vi "this application info.vi"(8 "error in":errorcluster, 11 "Build Type":enum16{"Release", "Patch", "Beta"}(ring)=enum."Patch") -> (0 "error out":errorcluster, 1 "App Info":T1, 2 "FileVersion":string, 3 "Title":string)   [LabVIEW 2020, in "Reusable Library.lvlib"]
doc: "This VI will return the Version info of the exe during runtime environment."
uses:
  Reusable Library.lvlib
panel:
  # "VI Template By\n        Samuel James\n        Measurement Engineer\n        Certified LabVIEW Architect\n        Vestas Technology R&D Chennai"
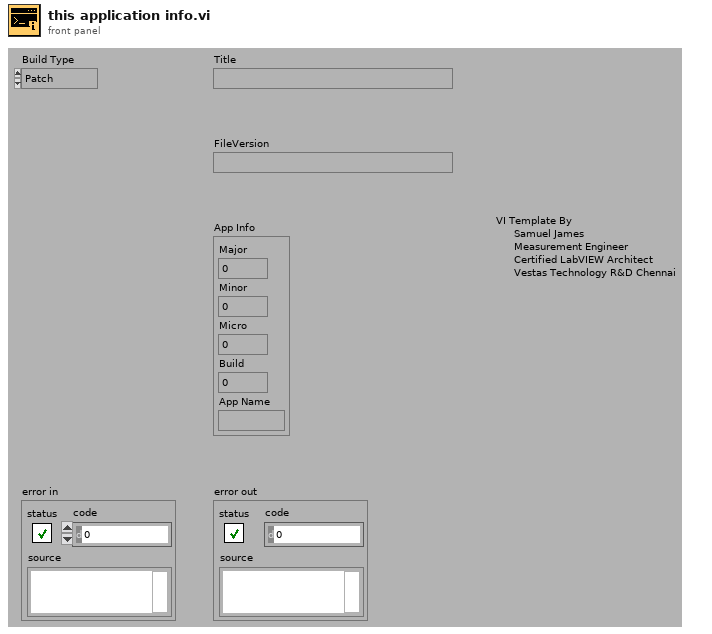
[diagram p1: front panel]
types:
  T1 = cluster{"Major":i32, "Minor":i32, "Micro":i32, "Build":i32, "App Name":string}
  T2 = enum32{"invalid app kind", "Development System", "Run Time System", "Student Edition", "Embedded LabVIEW", "Evaluation", "Custom"}
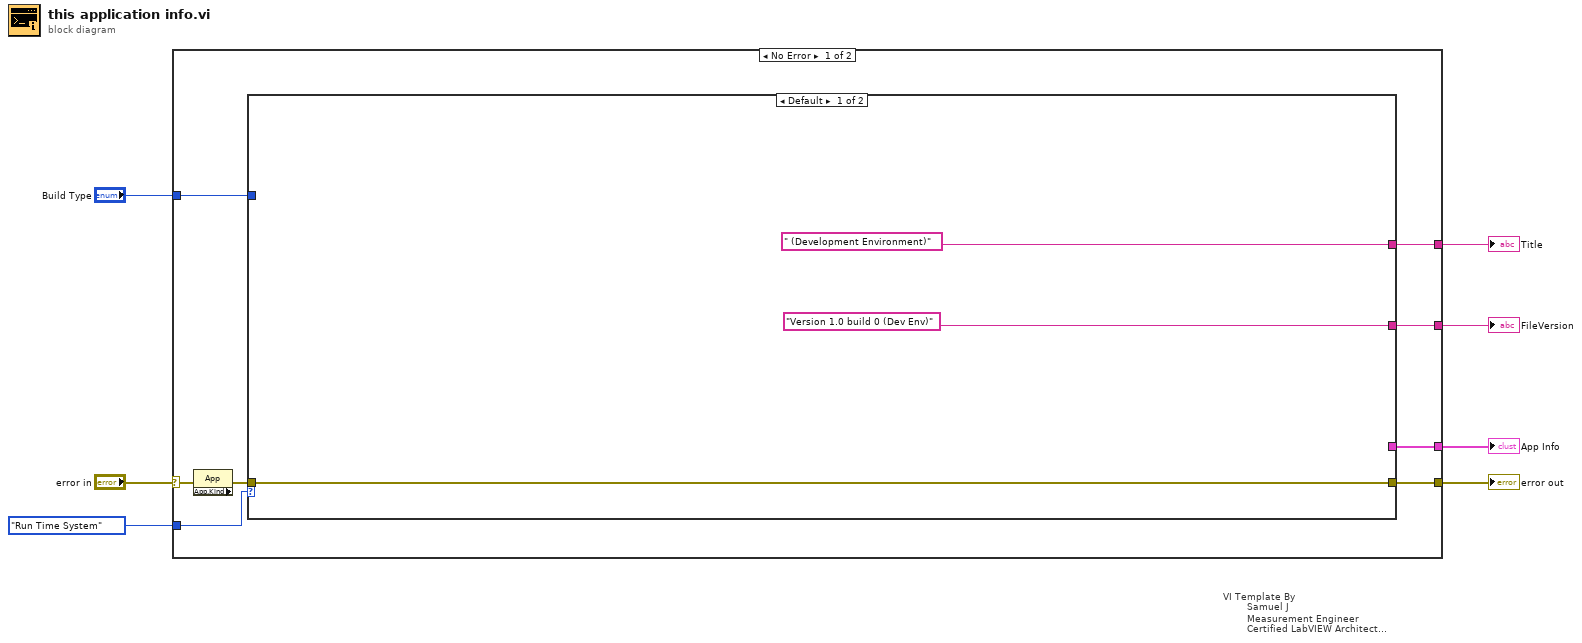
[diagram p0: block diagram]
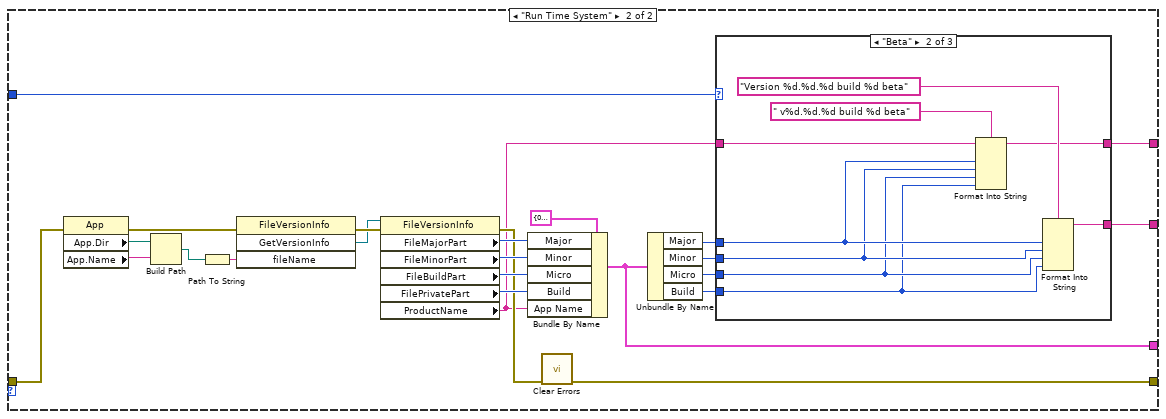
[diagram p2: hidden frame]
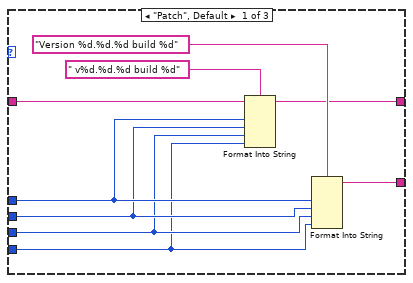
[diagram p3: hidden frame]
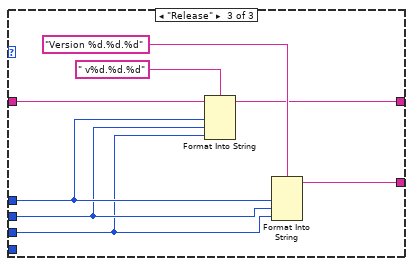
[diagram p4: hidden frame]
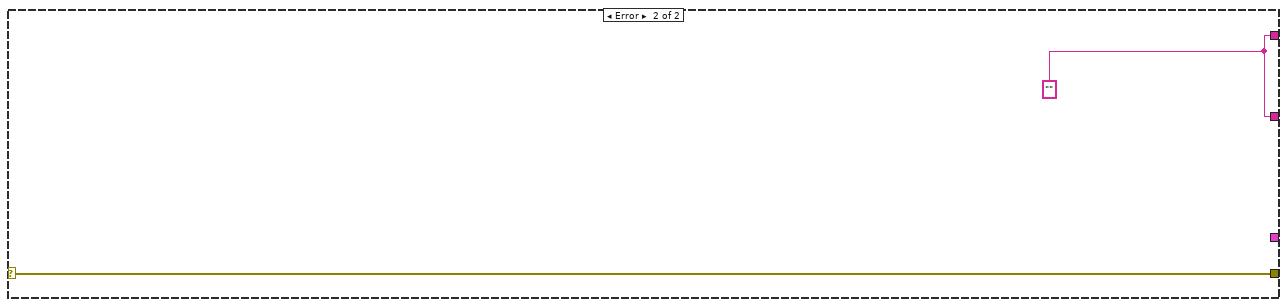
[diagram p5: hidden frame]
diagram:
  n1 = case "VI Template By\n        Samuel J\n        Measurement Engineer\n        Certified LabVIEW Architect\n        Vestas Technology R&D, Chennai" shown="No Error" "error in" {
    selector: "error in" -> [w11 w70]
    tunnel: [w15 w69] -> w7
    tunnel: [w14 w70] -> w5
    tunnel: [w12 w69] -> w4
    tunnel: T2."Run Time System" ("App.Kind") -> [w8 _]
    tunnel: "Build Type" -> [w10 _]
    tunnel: [w9 _] -> w1
    frame No Error {
      n2 = property class="App" props=["App.Kind"](error in=w11) -> (error out=w13:errorcluster)  [unwired: 1 in, 2 out]
      n3 = case shown="Default" w8 {
        tunnel: ["Version 1.0 build 0 (Dev Env)" w42] -> w15
        tunnel: [w18 w23] -> w14
        tunnel: w13 -> [w18 w40]
        tunnel: [" (Development Environment)" w41] -> w12
        tunnel: w10 -> [_ w28]
        tunnel: [_ w21] -> w9
        frame Default {
        }
        frame "Run Time System" {
          n4 = property class="App"(error in=w40) -> (error out=w39:errorcluster, "App.Dir"=w34:path, "App.Name"=w35:string)  [unwired: 1 in, 1 out]
          n5 = Build Path(base path=w34, name or relative path=w35) -> (appended path=w22:path)
          n6 = Path To String(path=w22) -> (string=w38:string)
          n7 = invoke class="FileVersionInfo" method="GetVersionInfo"(error in=w39, "fileName"=w38) -> (error out=w37:errorcluster, "GetVersionInfo"=w36:refnum<k24>)  [unwired: 2 in, 2 out]
          n8 = property class="FileVersionInfo"(reference=w36, error in=w37) -> (error out=w29:errorcluster, "FileMajorPart"=w33:i32, "FileMinorPart"=w32:i32, "FileBuildPart"=w31:i32, "FilePrivatePart"=w30:i32, "ProductName"=w19:string)  [unwired: 1 out]
          n9 = Bundle By Name(cluster=T1 {"Major"=0, "Minor"=0, "Micro"=0, "Build"=0, "App Name"=""} ("Cluster"), "Major"=w33, "Minor"=w32, "Micro"=w31, "Build"=w30, "App Name"=w19) -> (w21:T1)
          n10 = call <vilib>:"Clear Errors.vi"("error in (no error)"=w29) -> ("error out"=w23:errorcluster)  [unwired: 5 in, 1 out]
          n11 = Unbundle By Name(w21) -> ("Major"=w27:i32, "Minor"=w26:i32, "Micro"=w25:i32, "Build"=w24:i32)
          n12 = case shown="\"Beta\"" w28 {
            tunnel: [w50 w59 w67] -> w42
            tunnel: [w48 w57 w65] -> w41
            tunnel: w19 -> [w47 w56 w64]
            tunnel: w27 -> [w46 w55 w63]
            tunnel: w26 -> [w45 w54 w62]
            tunnel: w25 -> [w44 w53 w61]
            tunnel: w24 -> [w43 w52 _]
            frame "Patch", Default {
              n13 = Format Into String(format string=" v%d.%d.%d build %d", initial string=w47, w46, w45, w44, w43) -> (resulting string=w48:string)  [unwired: 1 in, 1 out]
              n14 = Format Into String(format string="Version %d.%d.%d build %d", w46, w45, w44, w43) -> (resulting string=w50:string)  [unwired: 2 in, 1 out]
            }
            frame "Beta" {
              n15 = Format Into String(format string=" v%d.%d.%d build %d beta", initial string=w56, w55, w54, w53, w52) -> (resulting string=w57:string)  [unwired: 1 in, 1 out]
              n16 = Format Into String(format string="Version %d.%d.%d build %d beta", w55, w54, w53, w52) -> (resulting string=w59:string)  [unwired: 2 in, 1 out]
            }
            frame "Release" {
              n17 = Format Into String(format string=" v%d.%d.%d", initial string=w64, w63, w62, w61) -> (resulting string=w65:string)  [unwired: 1 in, 1 out]
              n18 = Format Into String(format string="Version %d.%d.%d", w63, w62, w61) -> (resulting string=w67:string)  [unwired: 2 in, 1 out]
            }
          }
        }
      }
    }
    frame Error {
      w69 = ""
    }
  }
  "FileVersion" <- w7
  "error out" <- w5
  "Title" <- w4
  "App Info" <- w1
